vi "Parse Status Data.vi"(8 "error in":errorcluster, 11 "Data":string) -> (0 "error out":errorcluster, 1 "Status Explanation":string, 2 "Status String":string, 3 "Status":T1, 4 "Status Number":i32=-1)   [LabVIEW 2019, in "ACSVcontrol-driver.lvlib"]
doc: "Parse data recieved from PJVS with status."
uses:
  ACSVcontrol-driver.lvlib
  Type definitions/Status.ctl
  Type definitions/Status - Explanation.ctl
  <vilib>/Utility/error.llb/Error Cluster From Error Code.vi
  <vilib>/ErrorRing/Error Ring.xnode
panel:
  in  "Status (not input - only used as constant)":T1
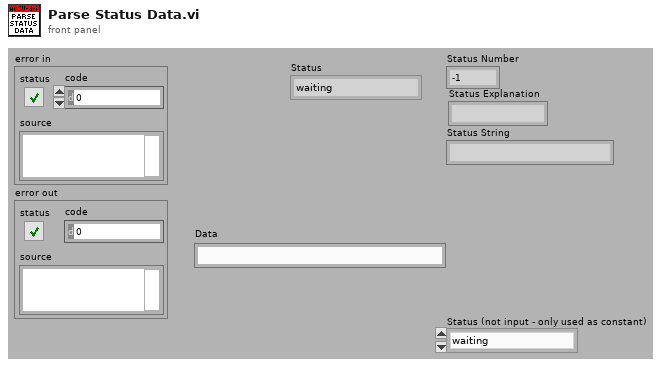
[diagram p1: front panel]
types:
  T1 = typedef "ACSVcontrol-driver.lvlib/Status.ctl" = enum16{"waiting", "processing", "error command", "Set_PJVS-Done", "Set_Mux-Done", "Set_Mux-Error", "Set_57XX-Done", "Set_57XX-Error", "Set_Gen-Done", "Set_Gen-Error", "Set_Synthesizer-Done", "Set_Synthesizer-Error", "Read_Nano-Done", "Read_Sampler-Done", "Read_Sampler-Error", "Read_Sensors-Done"}
  T2 = typedef "ACSVcontrol-driver.lvlib/Status - Explanation.ctl" = string[]
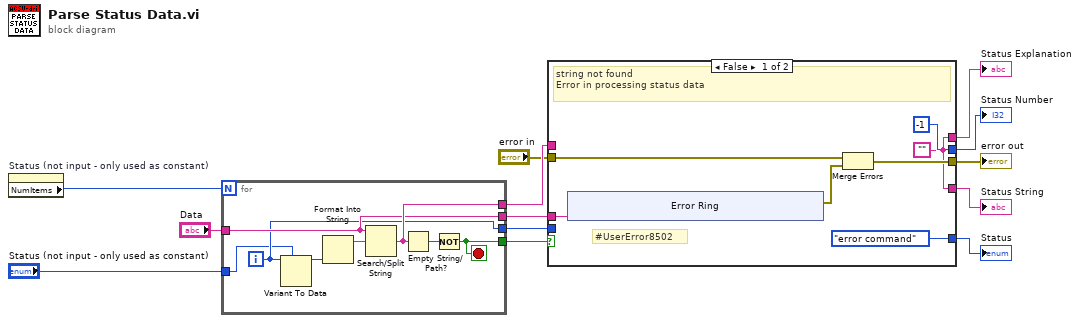
[diagram p0: block diagram]
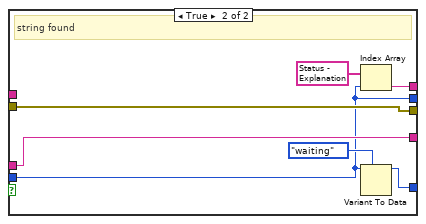
[diagram p2: hidden frame]
diagram:
  n1 = property on="Status (not input - only used as constant)" class="Enum (strict)"() -> ("NumItems"=w2:u32)  [unwired: 2 in, 2 out]
  n2 = for {
    N: w2 -> [_]
    tunnel: "Data" -> [w18]
    tunnel: [w20] -> w11
    tunnel: [w19] -> w12
    tunnel: [w16] -> w10
    tunnel: [w18] -> w9
    tunnel: "Status (not input - only used as constant)" -> [w14]
    i -> [w16]
    stop <- w19 stop-if-true
    n3 = Variant To Data(type=w14, Variant=w16) -> (data=w17:T1)  [unwired: 1 in, 1 out]
    n4 = Format Into String(w17) -> (resulting string=w15:string)  [unwired: 3 in, 1 out]
    n5 = Search/Split String(string=w18, search string/char (-)=w15) -> (match + rest of string=w20:string)  [unwired: 1 in, 2 out]
    n6 = Empty String/Path?(string/path=w20) -> (empty?=w21:bool)
    n7 = Not(x=w21) -> (.not. x?=w19:bool)
  }
  n8 = case shown="False" w12 {
    tunnel: w11 -> [_ _]
    tunnel: w10 -> [_ w37]
    tunnel: w9 -> [w27 w39]
    tunnel: [-1 w37] -> w8
    tunnel: [w23 w41] -> w7
    tunnel: [w25 w40] -> w6
    tunnel: "error in" -> [w26 w40]
    tunnel: [w23 w39] -> w4
    tunnel: [Status."error command" ("Status Data - Search Token") w36] -> w3
    frame False {
      w23 = ""
      # "#UserError8502"
      # "string not found\nError in processing status data"
      n9 = xnode "Error Ring"("parameter 0"=w27) -> ("error out"=w24:errorcluster)
      n10 = Merge Errors(w26, w24) -> (w25:errorcluster)
    }
    frame True {
      # "string found"
      n11 = Index Array(array=T2 ["AC-supraVOLTcontrol is waiting for a command to control something of the PJVS system.", "The software received the command and is processing the command at this time.", "There is some fault in the command, e.g. the length of the command is not correct, a parameter is missing or a parameter is out of the permissible range.", "The command Set_PJVS was executed successfully at the given time.", "The command Set_Mux wasn't executed successfully because of an error due to the communication with the multiplexer."] ("Status Data - Explanation"), index=w37) -> (element=w41:string)
      n12 = Variant To Data(type=Status."waiting" ("Status Data - Search Token"), Variant=w37) -> (data=w36:T1)  [unwired: 1 in, 1 out]
    }
  }
  "Status Number" <- w8
  "Status Explanation" <- w7
  "error out" <- w6
  "Status String" <- w4
  "Status" <- w3
